vi "Shoot.vi"   [LabVIEW 2019]
uses:
  <vilib>/Rock Robotics/WPI/ThirdParty/Phoenix-LabVIEW/Motor Controller/Controls/CTRE_Phoenix_MotorControl_ControlMode.ctl
types:
  T1 = typedef "WPI_MotorControlDeviceRef.ctl" = cluster{"DeviceStatus":errorcluster, "Type":T2, "PWM":cluster{"PWM Channel":T3, "DeadBand":T4}, "CAN":cluster{"Device Number":u8, "SetOutput VI Ref":variant, "GetOutput VI Ref":variant, "Enable VI Ref":variant, "Disable VI Ref":variant, "Data":variant}, "Invert":bool, "DIO PWM":cluster{"PWM \"Enable\" Channel":T3, "DIOChannel":T5, "PWM Rate":dbl}}
  T2 = typedef "WPI_MotorControlType.ctl" = enum16{"PWM", "CAN", "DIO PWM"}
  T3 = typedef "FPGA_DIOPWMChannel.ctl" = enum8{"PWM 0", "PWM 1", "PWM 2", "PWM 3", "PWM 4", "PWM 5", "PWM 6", "PWM 7", "PWM 8", "PWM 9", "PWM MXP 0", "PWM MXP 1", "PWM MXP 2", "PWM MXP 3", "PWM MXP 4", "PWM MXP 5", "PWM MXP 6", "PWM MXP 7", "PWM MXP 8", "PWM MXP 9", "Invalid"}
  T4 = typedef "WPI_PWMDeadband.ctl" = cluster{"Name":string, "maxPositivePwm":i32, "minPositivePwm":i32, "centerPwm":i32, "maxNegativePwm":i32, "minNegativePwm":i32, "angularRange":u16}
  T5 = typedef "FPGA_DIOChannel.ctl" = enum8{"DIO 0", "DIO 1", "DIO 2", "DIO 3", "DIO 4", "DIO 5", "DIO 6", "DIO 7", "DIO 8", "DIO 9", "DIO MXP 0", "DIO MXP 1", "DIO MXP 2", "DIO MXP 3", "DIO MXP 4", "DIO MXP 5", "DIO MXP 6", "DIO MXP 7", "DIO MXP 8", "DIO MXP 9", "DIO MXP 10", "DIO MXP 11", "DIO MXP 12", "DIO MXP 13", "DIO MXP 14", "DIO MXP 15", "SPI Port CS1", "SPI Port CS2", "SPI Port CS3", "SPI Port MISO", "SPI Port MOSI", "Invalid"}
  T6 = typedef "CTRE_Phoenix_MotorControl_ControlMode.ctl" = u16
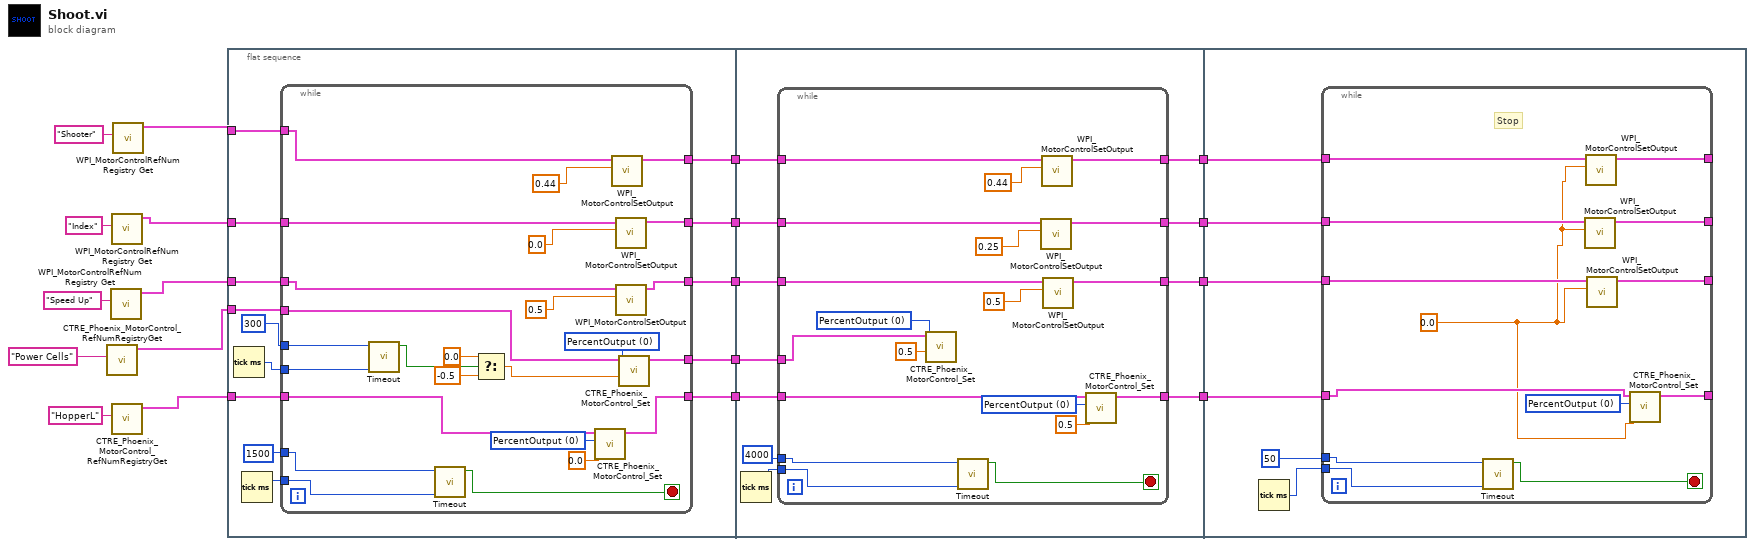
[diagram p0: block diagram]
diagram:
  n1 = call <vilib>:"CTRE_Phoenix_MotorControl_RefNumRegistryGet.vi"("refnum name"="Power Cells") -> ("PhoenixMotorControlDevRef"=w2:T1)  [unwired: 9 in, 1 out]
  n2 = call <vilib>:"WPI_MotorControlRefNum Registry Get.vi"("refnum name"="Speed Up") -> ("MotorControlDevRef"=w10:T1)  [unwired: 9 in, 1 out]
  n3 = call <vilib>:"WPI_MotorControlRefNum Registry Get.vi"("refnum name"="Index") -> ("MotorControlDevRef"=w11:T1)  [unwired: 9 in, 1 out]
  n4 = call <vilib>:"CTRE_Phoenix_MotorControl_RefNumRegistryGet.vi"("refnum name"="HopperL") -> ("PhoenixMotorControlDevRef"=w8:T1)  [unwired: 9 in, 1 out]
  n5 = call <vilib>:"WPI_MotorControlRefNum Registry Get.vi"("refnum name"="Shooter") -> ("MotorControlDevRef"=w15:T1)  [unwired: 9 in, 1 out]
  n6 = flat-sequence {
    tunnel: w15 -> [w33]
    tunnel: w11 -> [w31]
    tunnel: w10 -> [w30]
    tunnel: [w32] -> w19
    tunnel: [w29] -> w18
    tunnel: [w28] -> w17
    tunnel: w8 -> [w25]
    tunnel: [w24] -> w16
    tunnel: w2 -> [w21]
    tunnel: [w20] -> w1
    tunnel: w19 -> [w69]
    tunnel: w18 -> [w68]
    tunnel: w17 -> [w67]
    tunnel: w16 -> [w64]
    tunnel: [w63] -> w7
    tunnel: [w62] -> w6
    tunnel: [w61] -> w5
    tunnel: [w60] -> w4
    tunnel: w1 -> [w59]
    tunnel: w7 -> [w92]
    tunnel: w6 -> [w91]
    tunnel: w5 -> [w90]
    tunnel: w4 -> [w89]
    frame #0 {
      n7 = Tick Count (ms)() -> (millisecond timer value=w22:u32)
      n8 = Tick Count (ms)() -> (millisecond timer value=w27:u32)
      n9 = while {
        tunnel: w33 -> [w57]
        tunnel: [w58] -> w32
        tunnel: [w55] -> w29
        tunnel: w31 -> [w54]
        tunnel: [w52] -> w28
        tunnel: w30 -> [w50]
        tunnel: w27 -> [w44]
        tunnel: 1500 -> [w45]
        tunnel: w25 -> [w49]
        tunnel: [w46] -> w24
        tunnel: 300 -> [w42]
        tunnel: w22 -> [w41]
        tunnel: w21 -> [w39]
        tunnel: [w34] -> w20
        stop <- w43 stop-if-true
        w37 = T6 0 items=["PercentOutput"=0, "Position"=1, "Velocity"=2, "Current"=3, "Follower"=5, "MotionProfile"=6, "MotionMagic"=7, "MotionProfileArc"=10, "Disabled"=15] ("Control Mode")
        w48 = T6 0 items=["PercentOutput"=0, "Position"=1, "Velocity"=2, "Current"=3, "Follower"=5, "MotionProfile"=6, "MotionMagic"=7, "MotionProfileArc"=10, "Disabled"=15] ("Control Mode")
        n10 = call "Timeout.vi"("Start Time In"=w41, "Limit In"=w42) -> ("Timeout"=w40:bool)  [unwired: 8 in, 1 out]
        n11 = call "Timeout.vi"("Start Time In"=w44, "Limit In"=w45) -> ("Timeout"=w43:bool)  [unwired: 8 in, 1 out]
        n12 = Select(t=0.0, s=w40, f=-0.5) -> (s? t:f=w38:dbl)
        n13 = call <vilib>:"CTRE_Phoenix_MotorControl_Set.vi"("Output"=0.0, "Control Mode"=w48, "PhoenixMotorControlDevRef"=w49) -> ("PhoenixMotorControlDevRef"=w46:T1)  [unwired: 7 in, 1 out]
        n14 = call <vilib>:"WPI_MotorControlSetOutput.vi"("Output"=0.44, "MotorControlDevRef"=w57) -> ("MotorControlDevRef"=w58:T1)  [unwired: 7 in, 2 out]
        n15 = call <vilib>:"WPI_MotorControlSetOutput.vi"("Output"=0.0, "MotorControlDevRef"=w54) -> ("MotorControlDevRef"=w55:T1)  [unwired: 7 in, 2 out]
        n16 = call <vilib>:"WPI_MotorControlSetOutput.vi"("Output"=0.5, "MotorControlDevRef"=w50) -> ("MotorControlDevRef"=w52:T1)  [unwired: 7 in, 2 out]
        n17 = call <vilib>:"CTRE_Phoenix_MotorControl_Set.vi"("Output"=w38, "Control Mode"=w37, "PhoenixMotorControlDevRef"=w39) -> ("PhoenixMotorControlDevRef"=w34:T1)  [unwired: 7 in, 1 out]
      }
    }
    frame #1 {
      n18 = Tick Count (ms)() -> (millisecond timer value=w66:u32)
      n19 = while {
        tunnel: w69 -> [w88]
        tunnel: [w87] -> w60
        tunnel: [w86] -> w61
        tunnel: [w83] -> w62
        tunnel: w68 -> [w85]
        tunnel: w67 -> [w84]
        tunnel: w66 -> [w74]
        tunnel: 4000 -> [w75]
        tunnel: w64 -> [w77]
        tunnel: [w76] -> w63
        tunnel: w59 -> [w72]
        stop <- w73 stop-if-true
        w70 = T6 0 items=["PercentOutput"=0, "Position"=1, "Velocity"=2, "Current"=3, "Follower"=5, "MotionProfile"=6, "MotionMagic"=7, "MotionProfileArc"=10, "Disabled"=15] ("Control Mode")
        w79 = T6 0 items=["PercentOutput"=0, "Position"=1, "Velocity"=2, "Current"=3, "Follower"=5, "MotionProfile"=6, "MotionMagic"=7, "MotionProfileArc"=10, "Disabled"=15] ("Control Mode")
        n20 = call <vilib>:"CTRE_Phoenix_MotorControl_Set.vi"("Output"=0.5, "Control Mode"=w70, "PhoenixMotorControlDevRef"=w72) -> ()  [unwired: 7 in, 2 out]
        n21 = call "Timeout.vi"("Start Time In"=w74, "Limit In"=w75) -> ("Timeout"=w73:bool)  [unwired: 8 in, 1 out]
        n22 = call <vilib>:"WPI_MotorControlSetOutput.vi"("Output"=0.25, "MotorControlDevRef"=w85) -> ("MotorControlDevRef"=w86:T1)  [unwired: 7 in, 2 out]
        n23 = call <vilib>:"WPI_MotorControlSetOutput.vi"("Output"=0.44, "MotorControlDevRef"=w88) -> ("MotorControlDevRef"=w87:T1)  [unwired: 7 in, 2 out]
        n24 = call <vilib>:"WPI_MotorControlSetOutput.vi"("Output"=0.5, "MotorControlDevRef"=w84) -> ("MotorControlDevRef"=w83:T1)  [unwired: 7 in, 2 out]
        n25 = call <vilib>:"CTRE_Phoenix_MotorControl_Set.vi"("Output"=0.5, "Control Mode"=w79, "PhoenixMotorControlDevRef"=w77) -> ("PhoenixMotorControlDevRef"=w76:T1)  [unwired: 7 in, 1 out]
      }
    }
    frame #2 {
      n26 = Tick Count (ms)() -> (millisecond timer value=w94:u32)
      n27 = while {
        tunnel: w89 -> [w107]
        tunnel: [w106] -> _
        tunnel: [w105] -> _
        tunnel: [w102] -> _
        tunnel: w90 -> [w104]
        tunnel: w91 -> [w103]
        tunnel: w94 -> [w96]
        tunnel: 50 -> [w97]
        tunnel: w92 -> [w100]
        tunnel: [w99] -> _
        stop <- w95 stop-if-true
        w101 = T6 0 items=["PercentOutput"=0, "Position"=1, "Velocity"=2, "Current"=3, "Follower"=5, "MotionProfile"=6, "MotionMagic"=7, "MotionProfileArc"=10, "Disabled"=15] ("Control Mode")
        w98 = 0.0 ("Output")
        # "Stop"
        n28 = call "Timeout.vi"("Start Time In"=w96, "Limit In"=w97) -> ("Timeout"=w95:bool)  [unwired: 8 in, 1 out]
        n29 = call <vilib>:"WPI_MotorControlSetOutput.vi"("Output"=w98, "MotorControlDevRef"=w104) -> ("MotorControlDevRef"=w105:T1)  [unwired: 7 in, 2 out]
        n30 = call <vilib>:"WPI_MotorControlSetOutput.vi"("Output"=w98, "MotorControlDevRef"=w107) -> ("MotorControlDevRef"=w106:T1)  [unwired: 7 in, 2 out]
        n31 = call <vilib>:"WPI_MotorControlSetOutput.vi"("Output"=w98, "MotorControlDevRef"=w103) -> ("MotorControlDevRef"=w102:T1)  [unwired: 7 in, 2 out]
        n32 = call <vilib>:"CTRE_Phoenix_MotorControl_Set.vi"("Output"=w98, "Control Mode"=w101, "PhoenixMotorControlDevRef"=w100) -> ("PhoenixMotorControlDevRef"=w99:T1)  [unwired: 7 in, 1 out]
      }
    }
  }
